vi "ModbusDriverDataToServer.vi"(11 "DeviceListChannelData":T3) -> (3 "ServerData":T5, 5 "Status":T1[](array[typedef]))   [LabVIEW 2010]
uses:
  Ctrls/ServerData.ctl
  Ctrls/DeviceInfomation.ctl
  Ctrls/DeviceModel.ctl
  Ctrls/ChannelData.ctl
  Ctrls/ChannelType.ctl
  Ctrls/ChannelAccessType.ctl
  DeviceListChannelData.ctl
  AutoChannelData.ctl
  Ctrls/ConnectStatus.ctl
  MonitorServer.lvlib
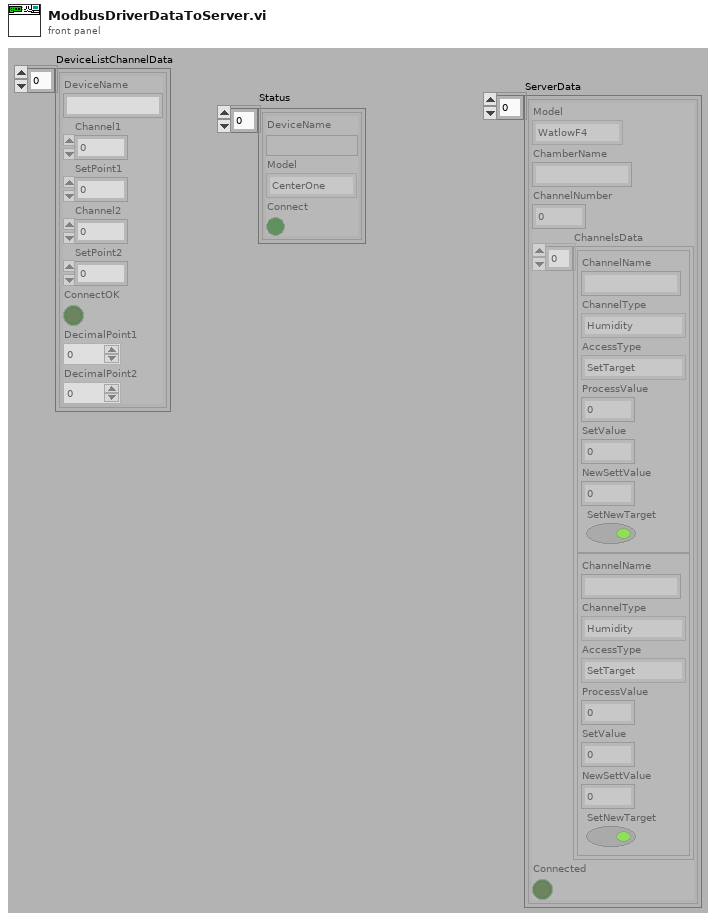
[diagram p1: front panel]
types:
  T1 = typedef "ConnectStatus.ctl" = cluster{"DeviceName":string, "Model":T2, "Connect":bool}
  T2 = typedef "DeviceModel.ctl" = enum16{"WatlowF4", "CenterOne", "DCP551", "DPR250"}
  T3 = typedef "MonitorServer.lvlib/DeviceListChannelData.ctl" = T4[]
  T4 = typedef "MonitorServer.lvlib/AutoChannelData.ctl" = cluster{"DeviceName":string, "Channel1":dbl, "SetPoint1":dbl, "Channel2":dbl, "SetPoint2":dbl, "ConnectOK":bool, "DecimalPoint1":i16, "DecimalPoint2":i16}
  T5 = typedef "ServerData.ctl" = T6[]
  T6 = typedef "DeviceInfomation.ctl" = cluster{"Model":T2, "ChamberName":string, "ChannelNumber":i32, "ChannelsData":T7[], "Connected":bool}
  T7 = typedef "ChannelData.ctl" = cluster{"ChannelName":string, "ChannelType":T8, "AccessType":T9, "ProcessValue":dbl, "SetValue":dbl, "NewSettValue":dbl, "SetNewTarget":bool}
  T8 = typedef "ChannelType.ctl" = enum16{"Temperature", "Humidity"}
  T9 = typedef "ChannelAccessType.ctl" = enum16{"ReadOnly", "SetTarget"}
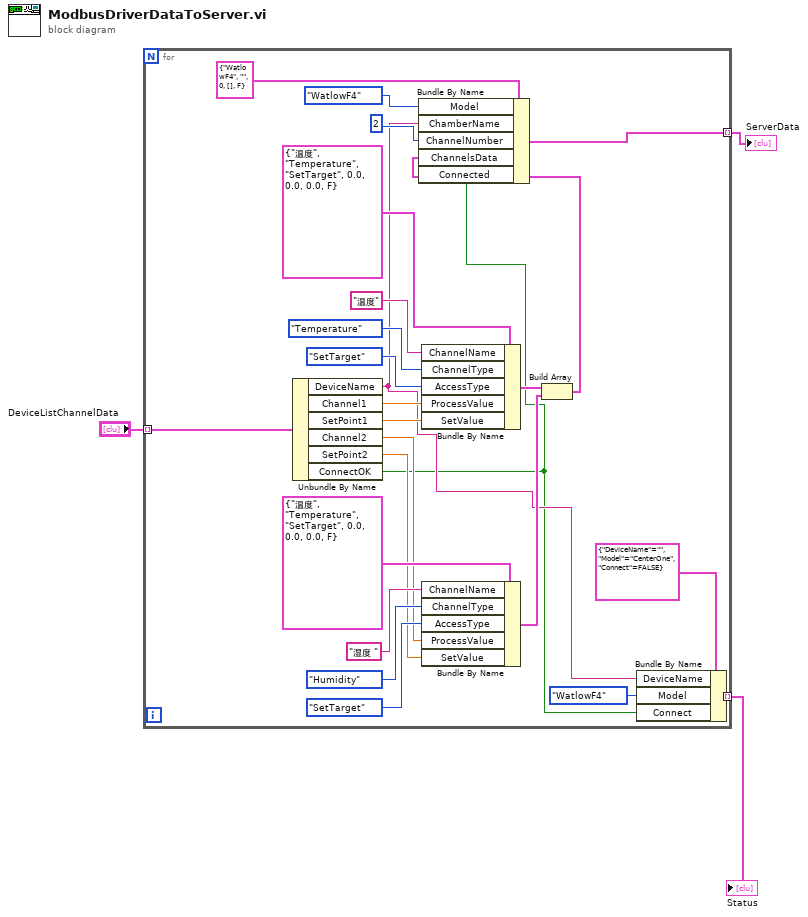
[diagram p0: block diagram]
diagram:
  n1 = for {
    tunnel: "DeviceListChannelData" -> [w28] mode=indexing
    tunnel: [w27] -> w2 mode=indexing
    tunnel: [w6] -> w1 mode=indexing
    n2 = Unbundle By Name(w28) -> ("DeviceName"=w8:string, "Channel1"=w20:dbl, "SetPoint1"=w19:dbl, "Channel2"=w12:dbl, "SetPoint2"=w11:dbl, "ConnectOK"=w4:bool)
    n3 = Bundle By Name(cluster=T7 {"ChannelName"="温度", "ChannelType"=enum."Temperature", "AccessType"=enum."SetTarget", "ProcessValue"=0.0, "SetValue"=0.0, "NewSettValue"=0.0, "SetNewTarget"=FALSE} ("ChannelInfomation"), "ChannelName"="温度", "ChannelType"=ChannelType."Temperature", "AccessType"=ChannelAccessType."SetTarget", "ProcessValue"=w20, "SetValue"=w19) -> (w18:T7)
    n4 = Bundle By Name(cluster=T7 {"ChannelName"="温度", "ChannelType"=enum."Temperature", "AccessType"=enum."SetTarget", "ProcessValue"=0.0, "SetValue"=0.0, "NewSettValue"=0.0, "SetNewTarget"=FALSE} ("ChannelInfomation"), "ChannelName"="湿度 ", "ChannelType"=ChannelType."Humidity", "AccessType"=ChannelAccessType."SetTarget", "ProcessValue"=w12, "SetValue"=w11) -> (w14:T7)
    n5 = Build Array(w18, w14) -> (w10:T7[])
    n6 = Bundle By Name(cluster=T6 {"Model"=enum."WatlowF4", "ChamberName"="", "ChannelNumber"=0, "ChannelsData"=[], "Connected"=FALSE} ("DeviceInfo"), "Model"=DeviceModel."WatlowF4", "ChamberName"=w8, "ChannelNumber"=2, "ChannelsData"=w10, "Connected"=w4) -> (w27:T6)
    n7 = Bundle By Name(cluster=T1 {"DeviceName"="", "Model"=enum."CenterOne", "Connect"=FALSE} ("ConnectStatus"), "DeviceName"=w8, "Model"=DeviceModel."WatlowF4", "Connect"=w4) -> (w6:T1)
  }
  "ServerData" <- w2
  "Status" <- w1
